vi "Configure Generation.vi"(8 "error in":errorcluster, 11 "AO DAQmx DC CFG in":refnum<class "AO DAQmx DC CFG.lvclass">) -> (0 "error out":errorcluster, 3 "AO DAQmx DC CFG out":refnum<class "AO DAQmx DC CFG.lvclass">)   [LabVIEW 2023, in "AO DAQmx DC CFG.lvclass"]
uses:
  AO DAQmx DC CFG.lvclass
  AO DAQmx DC CFG.lvclass/AO DAQmx DC CFG.ctl
  DAQmx/DAQmx Base CFG/DAQmx Base CFG.lvclass
  Configuration/Configuration JSON/Configuration JSON Base/CFG JSON.lvclass
  <vilib>/Utility/error.llb/Error Cluster From Error Code.vi
  <vilib>/ErrorRing/Error Ring.xnode
  <resource>/objmgr/daqmx.rc
  c67ae6e3-9b4c-4cdf-b959-69ccd0f59372.vi
  <vilib>/DAQmx/write.llb/DAQmx Write (Digital 1D Wfm NChan NSamp).vi
  D:/git/HAL/HAL GOOP4/DAQmx/DAQmx Base CFG/DAQmx Base CFG.lvclass
  D:/git/HAL/HAL GOOP4/CFG Target/CFG Target.lvclass
  D:/git/HAL/HAL GOOP4/Configuration/Configuration Semaphore/CFG Semaphore.lvclass
  D:/git/HAL/HAL GOOP4/Configuration/Configuration JSON/Configuration JSON Base/CFG JSON.lvclass
  D:/git/HAL/HAL GOOP4/Interfaces/IConfigure/IConfigure.lvclass
  D:/git/HAL/HAL GOOP4/AO/AO DAQmx DC CFG/AO DAQmx DC CFG.lvclass
  DAQmx/BufferWritesDBL/BufferWritesDBL.lvclass
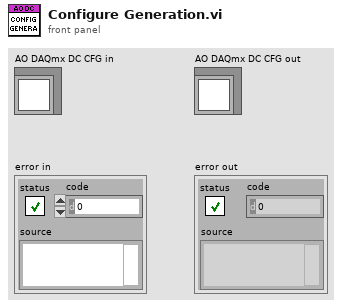
[diagram p1: front panel]
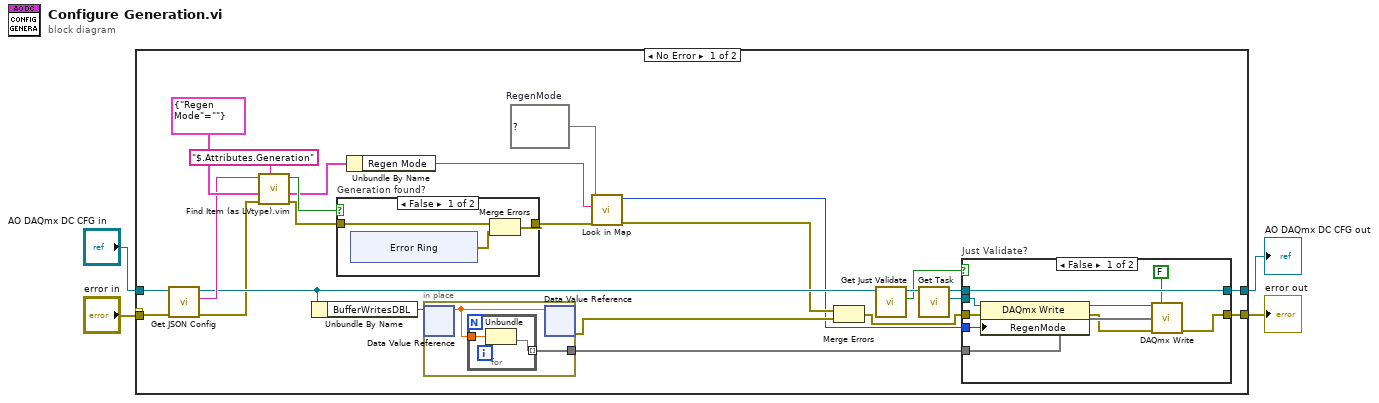
[diagram p0: block diagram]
diagram:
  n1 = case shown="No Error" {
    selector: _ -> [w10 w54]
    tunnel: [w16 w54] -> w1
    tunnel: [w17 w53] -> w2
    tunnel: "AO DAQmx DC CFG in" -> [w27 w53]
    tunnel: "error in" -> [_ _]
    frame No Error {
      w9 = map{string, i32} {"Allow Regeneration"=10097, "Do Not Allow Regeneration"=10158}  # RegenMode
      n2 = call "Get JSON Config.vi"("CFG Base in"=w27) -> ("<JSON>Config>"=w21:string, "CFG Base out"=w15:refnum<class "AO DAQmx DC CFG.lvclass">)  [unwired: 9 in]
      n3 = call "Find Item (as LVtype).vim"("$Path or Item Name"="$.Attributes.Generation", "error in (no error)"=w10, "Data Type and Default Value"=cluster{"Regen Mode":string} {"Regen Mode"=""}, "JSON"=w21) -> ("error out"=w26:errorcluster, "Data"=w22:cluster{"Regen Mode":string}, "Found"=w25:bool)  [unwired: 4 in, 1 out]
      n4 = Unbundle By Name(w15) -> ("BufferWritesDBL"=w14:refnum<class "BufferWritesDBL.lvclass">)
      n5 = case "Generation found?" shown="False" w25 {
        tunnel: w26 -> [w46 w52]
        tunnel: [w44 w52] -> w7
        frame False {
          n6 = xnode "Error Ring"() -> ("error out"=w45:errorcluster)
          n7 = Merge Errors(w46, w45) -> (w44:errorcluster)
        }
        frame True {
        }
      }
      n8 = Unbundle By Name(w22) -> ("Regen Mode"=w8:string)
      n9 = in-place {
        in-place-border: [w29] -> w13
        n10 = in-place-dvr #1(w14) -> (w30:dbl)  [unwired: 1 out]
        n11 = for {
          tunnel: w30 -> [w32]
          tunnel: [w31] -> w29 mode=indexing
          n12 = Unbundle(w32) -> (w31)  [unwired: 1 out]
        }
        n13 = in-place-dvr #1(w30) -> (w12:errorcluster)  [unwired: 1 out]
      }
      n14 = call "Look in Map.vi"("error in"=w7, "Key"=w8, "Map"=w9) -> ("error out"=w6:errorcluster, "Value"=w5:i32)  [unwired: 7 in]
      n15 = Merge Errors(w6, w12) -> (w11:errorcluster)
      n16 = call "Get Just Validate.vi"("CFG JSON Base in"=w15) -> ("Just Validate"=w19:bool, "CFG JSON Base out"=w20:refnum<class "AO DAQmx DC CFG.lvclass">)  [unwired: 9 in]
      n17 = call "Get Task.vi"("DAQmx Base CFG in"=w20) -> ("Task"=w28:refnum<k21>, "DAQmx Base CFG out"=w18:refnum<class "AO DAQmx DC CFG.lvclass">)  [unwired: 9 in]
      n18 = case "Just Validate?" shown="False" w19 {
        tunnel: w11 -> [w41 w42]
        tunnel: w28 -> [w40 _]
        tunnel: w5 -> [w39 _]
        tunnel: w18 -> [w34 w43]
        tunnel: [w34 w43] -> w17
        tunnel: [w35 w42] -> w16
        tunnel: w13 -> [w37 _]
        frame False {
          n19 = property class="DAQmx Write"(reference=w40, error in=w41, "RegenMode"=w39) -> (reference out=w38:refnum<k21>, error out=w36:errorcluster)
          n20 = call-poly <vilib>:"DAQmx Write.vi"("task/channels in"=w38, "auto start"=FALSE, "data"=w37, "error in"=w36) -> ("error out"=w35:errorcluster)  [unwired: 9 in, 2 out]
        }
        frame True {
        }
      }
    }
    frame Error {
    }
  }
  "error out" <- w1
  "AO DAQmx DC CFG out" <- w2
